vi "SVFA FFT Spectrum Subset (Mag-Phase).vi"   [LabVIEW 2017]
doc: "Computes a subset of the FFT spectrum of <B>scaled signal [EU]</B>. The subset is defined by <B>frequency range</B>. FFT results are returned as magnitude and phase. Each block of data corresponds to a single FFT block and has to be passed individually to this VI. Wire data to the <B>scaled signal [EU]</B> input to determine the polymorphic instance to use or manually select the instance."
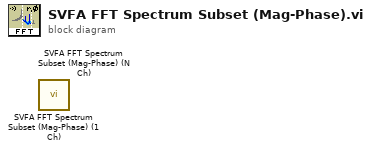
[diagram p0: block diagram]
diagram:
  n1 = call <vilib>:"SVFA FFT Spectrum Subset (Mag-Phase) (1 Ch).vi"() -> ()  [unwired: 12 in, 8 out]
  n2 = call <vilib>:"SVFA FFT Spectrum Subset (Mag-Phase) (N Ch).vi"() -> ()  [unwired: 12 in, 8 out]
